vi "Initialize Andor Camera.vi"() -> (0 "Error Out 2":errorcluster, 1 "Drv Success?":i32)   [LabVIEW 2014]
uses:
  Initilize Globals.vi
  lib/Andorlib/atmcd32d.lvlib
panel:
  out "Fastest VS Speed":sgl
  out "VS Speed":sgl[](array[numeric])
  out "pre-amp gains":sgl[](array[numeric])
  out "#preamp gains":i32
  out "# amplifiers":i32
  out "HS Speeds per channel":sgl[][](array[numeric])
  out "Bit Depth per channel":i32[](array[numeric])
  out "#ADC Channels":i32
  out "Lowest EM gain":i32
  out "Highest EM gain":i32
  out "Head Model":string
  out "eprom out":u32
  out "Camera Serial #":i32
  out "PCB version #":u32
  out "Directory Out":string
  out "Camera FirmWare Version":i32
  out "Y-pixels":u32
  out "X-pixels":u32
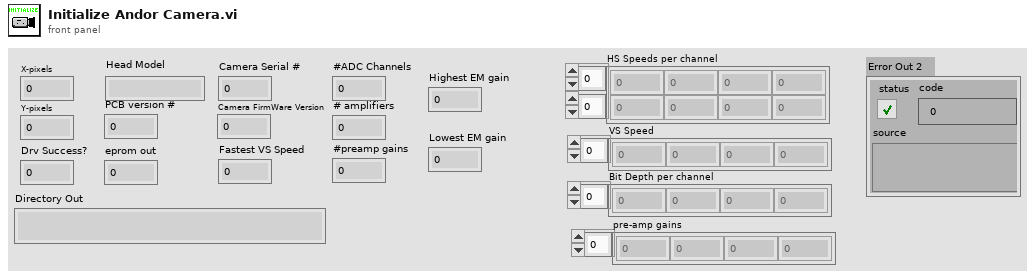
[diagram p1: front panel]
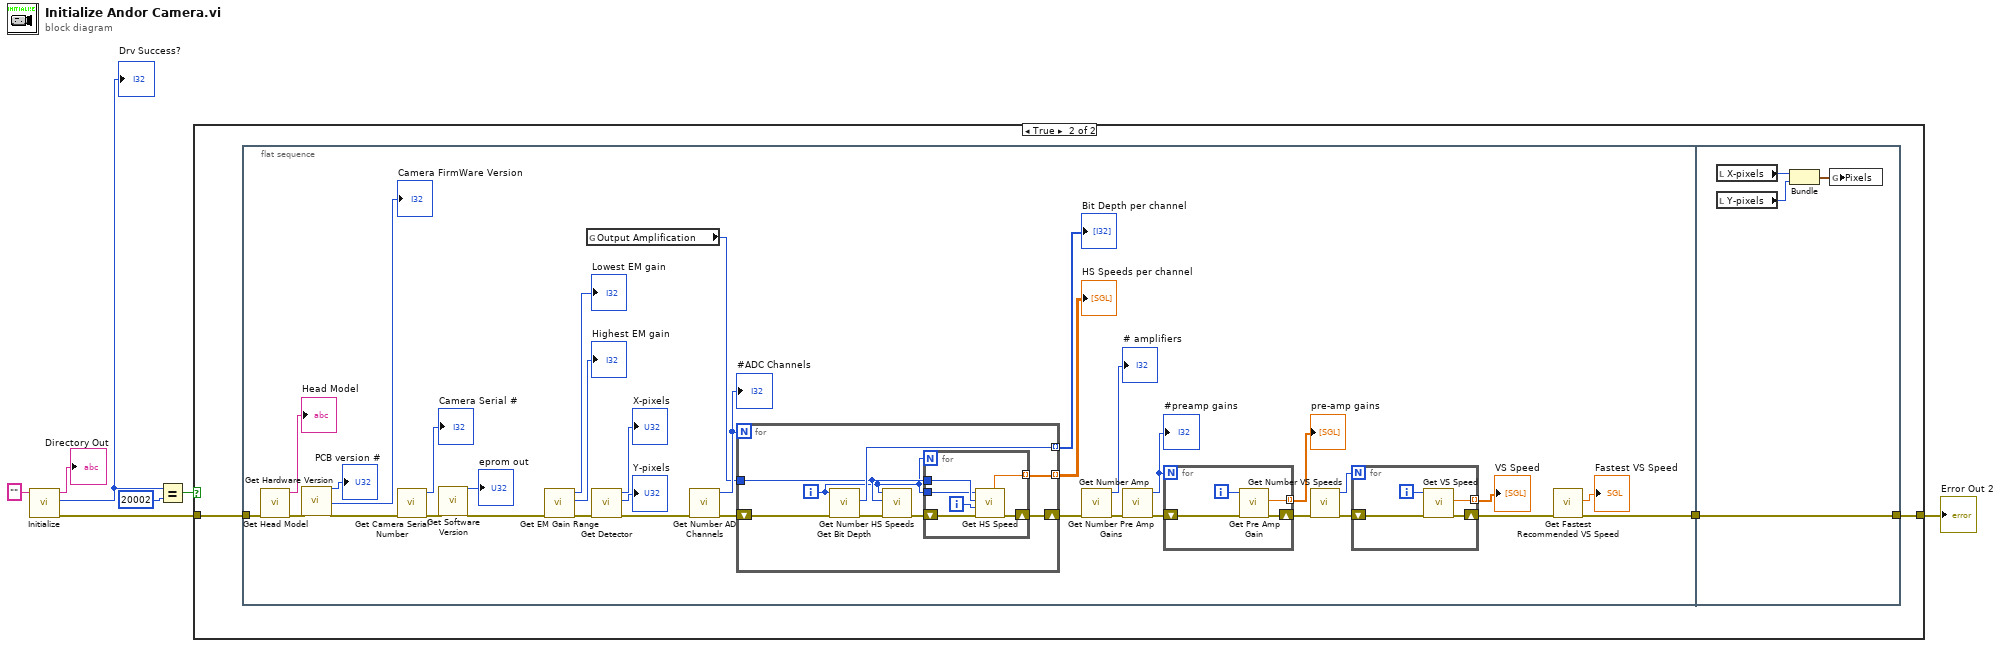
[diagram p0: block diagram]
diagram:
  n1 = call "Initialize.vi"("dir"="") -> ("error out"=w6:errorcluster, "function return"=w2:u32, "dir out"=→"Directory Out":string)  [unwired: 8 in]
  "Drv Success?" <- w2
  n2 = Equal?(x=w2, y=20002) -> (x = y?=w3:bool)
  n3 = case shown="True" w3 {
    tunnel: [w8 w9] -> w7
    tunnel: w6 -> [w8 w11]
    frame False {
    }
    frame True {
      n4 = flat-sequence {
        tunnel: w11 -> [w37]
        tunnel: [w12] -> w10
        tunnel: [w68] -> w9
        tunnel: w10 -> [w68]
        frame #0 {
          n5 = call "Get Head Model.vi"("error in (no error)"=w37) -> ("error out"=w35:errorcluster, "name out"=→"Head Model":string)  [unwired: 8 in, 1 out]
          n6 = call "Get Hardware Version.vi"("error in (no error)"=w35) -> ("PCB out"=→"PCB version #":u32, "CameraFirmwareVersion out"=→"Camera FirmWare Version":u32, "error out"=w41:errorcluster)  [unwired: 19 in, 5 out]
          n7 = call "Get Camera Serial Number.vi"("error in (no error)"=w41) -> ("error out"=w39:errorcluster, "number out"=→"Camera Serial #":i32)  [unwired: 8 in, 1 out]
          n8 = call "Get Software Version.vi"("error in (no error)"=w39) -> ("eprom out"=→"eprom out":u32, "error out"=w33:errorcluster)  [unwired: 19 in, 6 out]
          n9 = call "Get EM Gain Range.vi"("error in (no error)"=w33) -> ("error out"=w32:errorcluster, "high out"=→"Highest EM gain":i32, "low out"=→"Lowest EM gain":i32)  [unwired: 7 in, 1 out]
          n10 = global read "Initilize Globals.vi" "Output Amplification"() -> (w26:i32)
          n11 = call "Get Detector.vi"("error in (no error)"=w32) -> ("error out"=w34:errorcluster, "ypixels out"=→"Y-pixels":i32, "xpixels out"=→"X-pixels":i32)  [unwired: 7 in, 1 out]
          n12 = call "Get Number AD Channels.vi"("error in (no error)"=w34) -> ("error out"=w28:errorcluster, "channels out"=w29:i32)  [unwired: 8 in, 1 out]
          "#ADC Channels" <- w29
          n13 = for {
            N: w29 -> [_]
            shift-right: [w57] -> w24
            shift-left: w28 -> [w61]
            tunnel: [w60] -> w27 mode=indexing
            tunnel: w26 -> [w55]
            tunnel: [w56] -> w25 mode=indexing
            i -> [w54]
            n14 = call "Get Bit Depth.vi"("error in (no error)"=w61, "channel"=w54) -> ("error out"=w59:errorcluster, "depth out"=w60:i32)  [unwired: 7 in, 1 out]
            n15 = call "Get Number HS Speeds.vi"("error in (no error)"=w59, "typ"=w55, "channel"=w54) -> ("error out"=w58:errorcluster)  [unwired: 6 in, 2 out]
            n16 = for {
              N: w54 -> [_]
              shift-right: [w65] -> w57
              shift-left: w58 -> [w66]
              tunnel: [w64] -> w56 mode=indexing
              tunnel: w55 -> [w63]
              tunnel: w54 -> [w62]
              i -> [w67]
              n17 = call "Get HS Speed.vi"("error in (no error)"=w66, "index"=w67, "typ"=w63, "channel"=w62) -> ("error out"=w65:errorcluster, "speed out"=w64:sgl)  [unwired: 5 in, 1 out]
            }
          }
          "Bit Depth per channel" <- w27
          "HS Speeds per channel" <- w25
          n18 = call "Get Number Amp.vi"("error in (no error)"=w24) -> ("error out"=w22:errorcluster, "amp out"=→"# amplifiers":i32)  [unwired: 8 in, 1 out]
          n19 = call "Get Number Pre Amp Gains.vi"("error in (no error)"=w22) -> ("error out"=w21:errorcluster, "noGains out"=w20:i32)  [unwired: 8 in, 1 out]
          "#preamp gains" <- w20
          n20 = for {
            N: w20 -> [_]
            shift-right: [w52] -> w18
            shift-left: w21 -> [w53]
            tunnel: [w50] -> w19 mode=indexing
            i -> [w51]
            n21 = call "Get Pre Amp Gain.vi"("error in (no error)"=w53, "index"=w51) -> ("error out"=w52:errorcluster, "gain out"=w50:sgl)  [unwired: 7 in, 1 out]
          }
          "pre-amp gains" <- w19
          n22 = call "Get Number VS Speeds.vi"("error in (no error)"=w18) -> ("error out"=w17:errorcluster, "speeds out"=w16:i32)  [unwired: 8 in, 1 out]
          n23 = for {
            N: w16 -> [_]
            shift-right: [w48] -> w14
            shift-left: w17 -> [w49]
            tunnel: [w46] -> w15 mode=indexing
            i -> [w47]
            n24 = call "Get VS Speed.vi"("error in (no error)"=w49, "index"=w47) -> ("error out"=w48:errorcluster, "speed out"=w46:sgl)  [unwired: 7 in, 1 out]
          }
          "VS Speed" <- w15
          n25 = call "Get Fastest Recommended VS Speed.vi"("error in (no error)"=w14) -> ("error out"=w12:errorcluster, "speed out"=→"Fastest VS Speed":sgl)  [unwired: 7 in, 2 out]
        }
        frame #1 {
          n26 = local read "X-pixels"() -> (w70:u32)
          n27 = local read "Y-pixels"() -> (w69:u32)
          n28 = Bundle("X-pixels"=w70, "Y-pixels"=w69) -> (w71:cluster{"X-pixels":u32, "Y-pixels":u32})  [unwired: 1 in]
          n29 = global write "Initilize Globals.vi" "Pixels"(w71) -> ()
        }
      }
    }
  }
  "Error Out 2" <- w7
